vi "IT8800-Query Range Limit.vi"(8 "error in":errorcluster, 10 "Range Type":T2, 11 "IT8800 Setting In In":T1={"VISA Resource Name"="", "Baud Rate"=19200, "Stop Bits"=20, "Wait For Read(ms)"=0, "Interface Type"=enum."VXI", "Limits"=[]} {"Stop Bits" items=["1.0"=10, "2.0"=20]; "Baud Rate" items=["2400"=2400, "4800"=4800, "9600"=9600, "19200"=19200]}) -> (0 "error out":errorcluster, 2 "Range":dbl, 3 "IT8800 Setting In Out":T1={"VISA Resource Name"="", "Baud Rate"=19200, "Stop Bits"=20, "Wait For Read(ms)"=0, "Interface Type"=enum."VXI", "Limits"=[]} {"Stop Bits" items=["1.0"=10, "2.0"=20]; "Baud Rate" items=["2400"=2400, "4800"=4800, "9600"=9600, "19200"=19200]})   [LabVIEW 2018]
uses:
  Data Def/IT8800-Operation Mode.ctl
  Data Def/IT8800-Setting.ctl
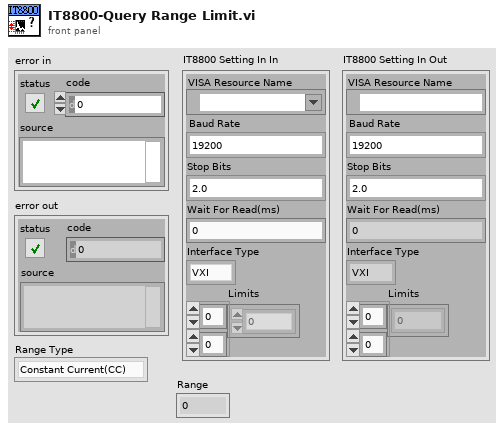
[diagram p1: front panel]
types:
  T1 = typedef "IT8800-Setting.ctl" = cluster{"VISA Resource Name":refnum<visa-resource-name>, "Baud Rate":u32, "Stop Bits":u16, "Wait For Read(ms)":u32, "Interface Type":enum16{"Unknow", "GPIB", "VXI", "GPIB-VXI", "Serial", "PXI", "TCPIP", "USB", "FireWire"}, "Limits":dbl[][]}
  T2 = typedef "IT8800-Operation Mode.ctl" = enum16{"Constant Current(CC)", "Constant Voltage(CV)", "Constant Power(CP)", "Constant Resistance(CR)"}
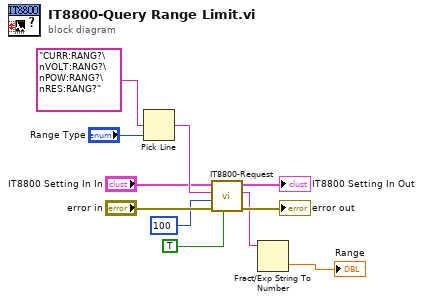
[diagram p0: block diagram]
diagram:
  n1 = Pick Line(multi-line string="CURR:RANG?\nVOLT:RANG?\nPOW:RANG?\nRES:RANG?", line index="Range Type") -> (output string=w5:string)  [unwired: 1 in]
  n2 = call "IT8800-Request.vi"("Response?"=TRUE, "error in"="error in", "byte count"=u32 100, "Command"=w5, "IT8800 Setting In In"="IT8800 Setting In In") -> ("error out"=→"error out":errorcluster, "Response"=w4:string, "IT8800 Setting In Out"=→"IT8800 Setting In Out":T1)  [unwired: 4 in]
  n3 = Fract/Exp String To Number(string=w4) -> (number=→"Range":dbl)  [unwired: 3 in, 1 out]
